vi "MainCamera_simulation.vi"() -> ()   [LabVIEW 2018]
uses:
  <vilib>/addons/lvgpu/lvcufft/CUFFT Type (cufftType).ctl
  <vilib>/Analysis/baseanly.llb/Real Outer Product.vi
  <vilib>/addons/lvgpu/lvcufft/Create 2D FFT Plan.vi
  <vilib>/Analysis/Matrix/Numeric/Conversions/Matrix To Array - RM.vi
  <vilib>/measure/NI_MABase.lvlib
  <vilib>/Analysis/NI_AALBase.lvlib
  <vilib>/Analysis/Matrix/NI_Matrix.lvlib
  <vilib>/addons/lvgpu/lvcuda.lvlib
  <vilib>/addons/lvgpu/lvcufft.lvlib
panel:
  out "size(s)":i32[](array[numeric])
  out "error out":errorcluster
  out "Intensity Graph":dbl[][](graph)
  in  "noise amplitude":dbl=0.1 format="%#.6g"
  in  "noise type":T1(ring)=enum."inverse f"
  out "Waveform Graph":waveform(dbl)(graph)
  in  "Stop":bool
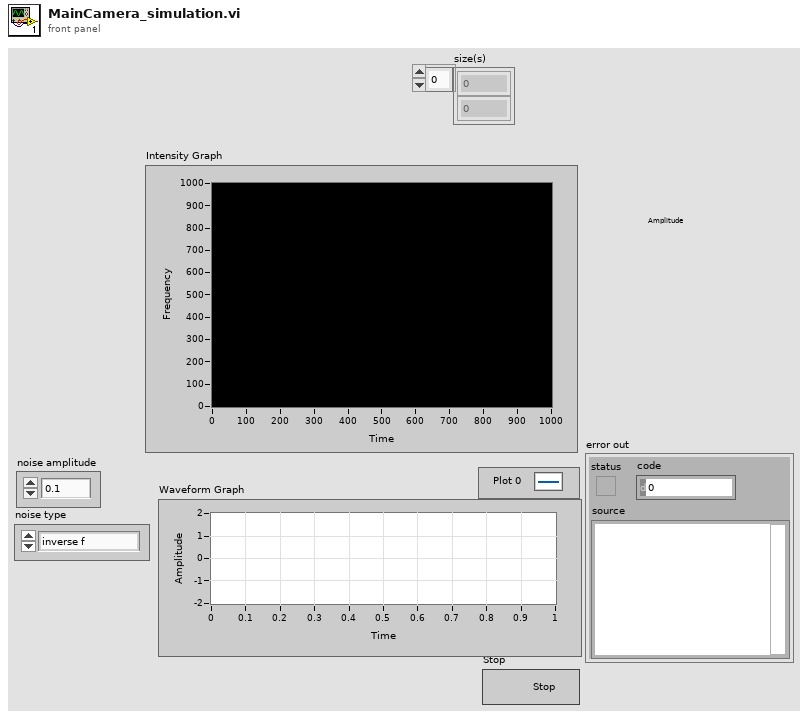
[diagram p1: front panel]
types:
  T1 = enum16{"uniform white", "Gaussian white", "periodic", "inverse f"}
  T2 = typedef "lvcufft.lvlib/CUFFT Type (cufftType).ctl" = i32
  T3 = cluster{"lower cutoff freq":dbl, "higher cutoff freq":dbl, "order":i32}
  T4 = typedef "NI_Matrix.lvlib/RealMatrix.ctl" = dbl[][]
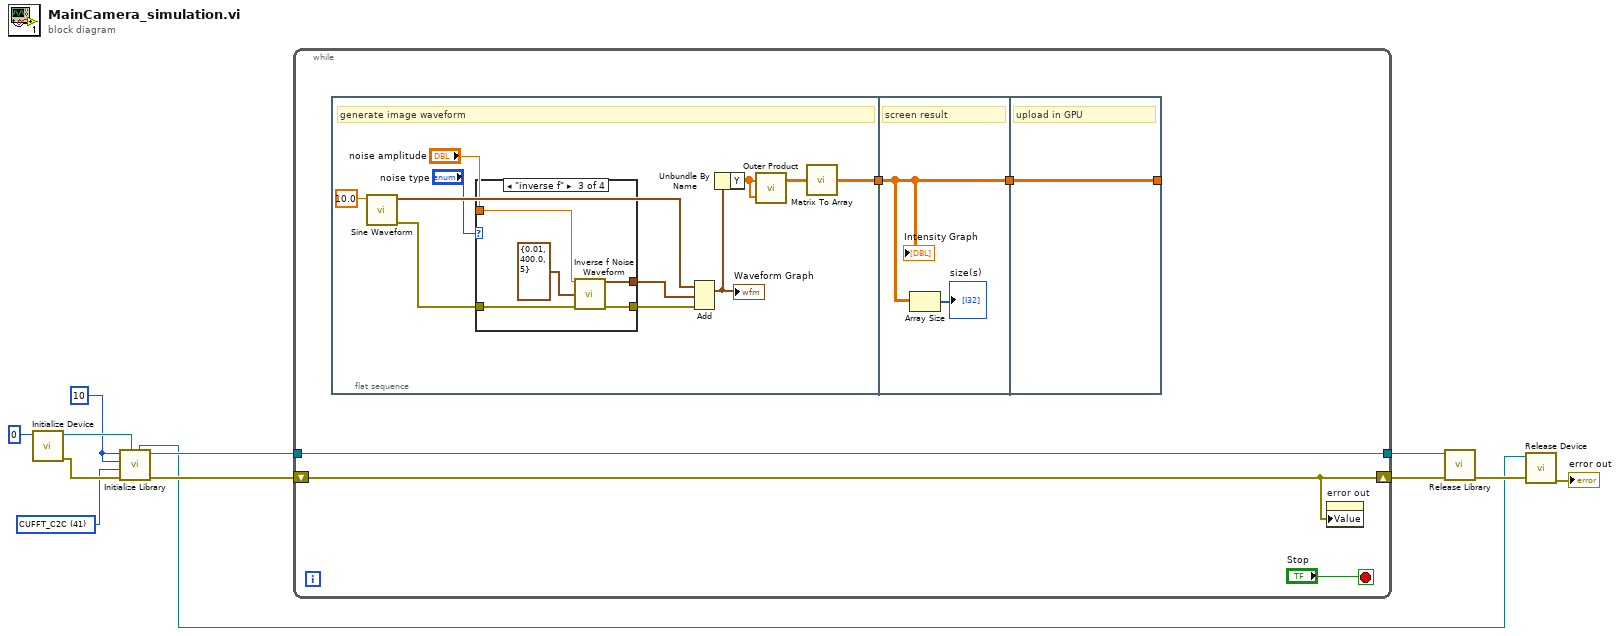
[diagram p0: block diagram]
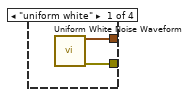
[diagram p2: hidden frame]
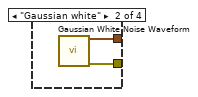
[diagram p3: hidden frame]
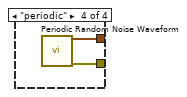
[diagram p4: hidden frame]
diagram:
  w4 = T2 41 items=["CUFFT_R2C"=42, "CUFFT_C2R"=44, "CUFFT_C2C"=41, "CUFFT_D2Z"=106, "CUFFT_Z2D"=108, "CUFFT_Z2Z"=105] ("type")
  w5 = 10
  n1 = call <vilib>:"Initialize Device.vi"("CUDA Device ID"=0) -> ("error out"=w10:errorcluster, "CUDA Context"=w11:refnum<class "CUDA Context.lvclass">)  [unwired: 8 in, 1 out]
  n2 = call-poly <vilib>:"Initialize Library.vi"("CUDA Context in"=w11, "error in"=w10, "type"=w4, "columns"=w5, "rows"=w5) -> ("error out"=w9:errorcluster, "CUFFT Handle"=w7:refnum<class "CUFFT Handle.lvclass">, "CUDA Context out"=w2:refnum<class "CUDA Context.lvclass">)  [unwired: 3 in, 1 out]
  n3 = while {
    tunnel: w7 -> [w14]
    tunnel: [w14] -> w6
    shift-right: [w13] -> w8
    shift-left: w9 -> [w13]
    stop <- "Stop" stop-if-true
    n4 = flat-sequence {
      tunnel: [w18] -> w16
      tunnel: w16 -> [w41]
      tunnel: [w41] -> w15
      tunnel: [w42] -> _
      tunnel: w15 -> [w42]
      frame #0 {
        # "generate image waveform"
        n5 = call <vilib>:"Sine Waveform.vi"("frequency"=10.0) -> ("error out"=w24:errorcluster, "signal out"=w26:waveform(dbl))  [unwired: 9 in]
        n6 = case shown="\"inverse f\"" "noise type" {
          tunnel: [w30 w32 w37 w39] -> w25
          tunnel: [w29 w31 w36 w38] -> w22
          tunnel: w24 -> [_ _ w34 _]
          tunnel: "noise amplitude" -> [_ _ w33 _]
          frame "uniform white" {
            n7 = call <vilib>:"Uniform White Noise Waveform.vi"() -> ("error out"=w29:errorcluster, "signal out"=w30:waveform(dbl))  [unwired: 10 in]
          }
          frame "Gaussian white" {
            n8 = call <vilib>:"Gaussian White Noise Waveform.vi"() -> ("error out"=w31:errorcluster, "signal out"=w32:waveform(dbl))  [unwired: 10 in]
          }
          frame "inverse f" {
            n9 = call <vilib>:"Inverse f Noise Waveform.vi"("noise density"=w33, "filter specifications"=T3 {"lower cutoff freq"=0.01, "higher cutoff freq"=400.0, "order"=5}, "error in (no error)"=w34) -> ("signal out"=w37:waveform(dbl), "error out"=w36:errorcluster)  [unwired: 8 in, 3 out]
          }
          frame "periodic" {
            n10 = call <vilib>:"Periodic Random Noise Waveform.vi"() -> ("error out"=w38:errorcluster, "signal out"=w39:waveform(dbl))  [unwired: 10 in]
          }
        }
        n11 = Add(1:w25, 2:w26, 4:w22) -> (0:w21:waveform(dbl))  [unwired: 1 out]
        "Waveform Graph" <- w21
        n12 = Unbundle By Name(w21) -> ("Y"=w27:dbl[])
        n13 = call-poly <vilib>:"Outer Product.vi"("Y Vector"=w27, "X Vector"=w27) -> ("Outer Product"=w20:T4)  [unwired: 1 out]
        n14 = call-poly <vilib>:"Matrix To Array.vi"("Real Matrix"=w20) -> ("Real 2D Array"=w18:dbl[][])
      }
      frame #1 {
        # "screen result"
        n15 = Array Size(array=w41) -> (size(s)=→"size(s)":i32[])
        "Intensity Graph" <- w41
      }
      frame #2 {
        # "upload in GPU"
      }
    }
    n16 = property on="error out" class="Clust (strict)"("Value"=w13) -> ()  [unwired: 2 in, 2 out]
  }
  n17 = call <vilib>:"Release Library.vi"("error in"=w8, "CUFFT Handle in"=w6) -> ("error out"=w3:errorcluster)  [unwired: 9 in]
  n18 = call <vilib>:"Release Device.vi"("error in"=w3, "CUDA Context in"=w2) -> ("error out"=→"error out":errorcluster)  [unwired: 9 in]
